vi "CorrectMoveAngleSign.vi"(10 "Direction":bool, 11 "Step size (deg) in":dbl) -> (3 "Step size (deg) out":dbl)   [LabVIEW 2013]
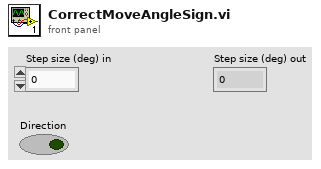
[diagram p1: front panel]
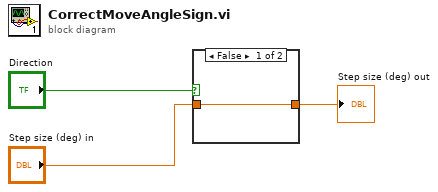
[diagram p0: block diagram]
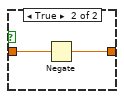
[diagram p2: hidden frame]
diagram:
  n1 = case shown="False" "Direction" {
    tunnel: "Step size (deg) in" -> [w4 w6]
    tunnel: [w4 w5] -> w3
    frame False {
    }
    frame True {
      n2 = Negate(x=w6) -> (-x=w5:dbl)
    }
  }
  "Step size (deg) out" <- w3
